vi "PreprocessMotorStages.vi"(3 "Speed Regulation":bool, 5 "Wait":bool=TRUE, 6 "Direction (T: Fwd)":bool=TRUE, 7 "Stop After":bool=TRUE, 8 "Power":i32=75, 9 "Ramp Mode":T5 items=["Constant", "Ramp Up", "Ramp Down"], 10 "Goal":i32=360, 11 "Goal Type":T4=1 items=["Unlimited", "Distance", "Time", "Stop"]) -> (1 "stages":i32=2, 2 "stage definitions":T1[](array[typedef])=[{"Power"=75, "Mode"=3, "RegMode"=0, "RunState"=32, "Goal Type"=1, "Goal"=360, "Update Flags"=39}, {"Power"=0, "Mode"=7, "RegMode"=1, "RunState"=32, "Goal Type"=3, "Goal"=500, "Update Flags"=7}] {"Update Flags" format="%.0x"; "Goal Type" items=["Unlimited", "Distance", "Time", "Stop"]; "RunState" format="%02.0f" items=["IDLE"=0, "RAMPUP"=16, "RUNNING"=32, "RAMPDOWN"=64]; "RegMode" format="%02.0f" items=["IDLE", "SPEED", "SYNC"]; "Mode" format="%.0x"})   [LabVIEW 2009]
uses:
  <vilib>/NXT/Block Support/NXT_Motor.Action.ctl
  <vilib>/NXT/Block Support/NXT_OutputGoalType.ctl
  MotorStageDefinition.ctl
  Move/RegMode.ctl
  Move/RunState.ctl
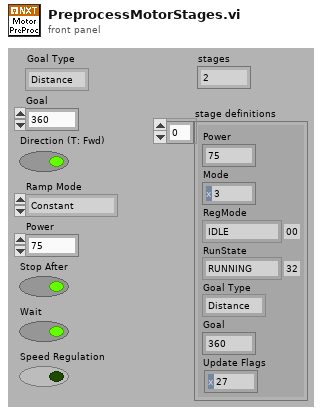
[diagram p1: front panel]
types:
  T1 = typedef "MotorStageDefinition.ctl" = cluster{"Power":i8, "Mode":u8, "RegMode":T2, "RunState":T3, "Goal Type":T4, "Goal":u32, "Update Flags":u8}
  T2 = typedef "RegMode.ctl" = u8
  T3 = typedef "RunState.ctl" = u8
  T4 = typedef "NXT_OutputGoalType.ctl" = u16
  T5 = typedef "NXT_Motor.Action.ctl" = u16
  T6 = cluster{i8, u8, "RegMode":T2, "RunState":T3, "Goal Type":T4, "Goal":u32, u8}
  T7 = cluster{i8, u8, "RegMode":T2, "RunState":T3, u8, "Absolute Value":i32, u8}
  T8 = cluster{i8, u8, "RegMode":T2, "RunState":T3, u8, "Absolute Value":i32, u8}[]
  T9 = cluster{i8, u8, "RegMode":T2, "RunState":T3, "Goal Type":T4, "Goal":u32, u8}[]
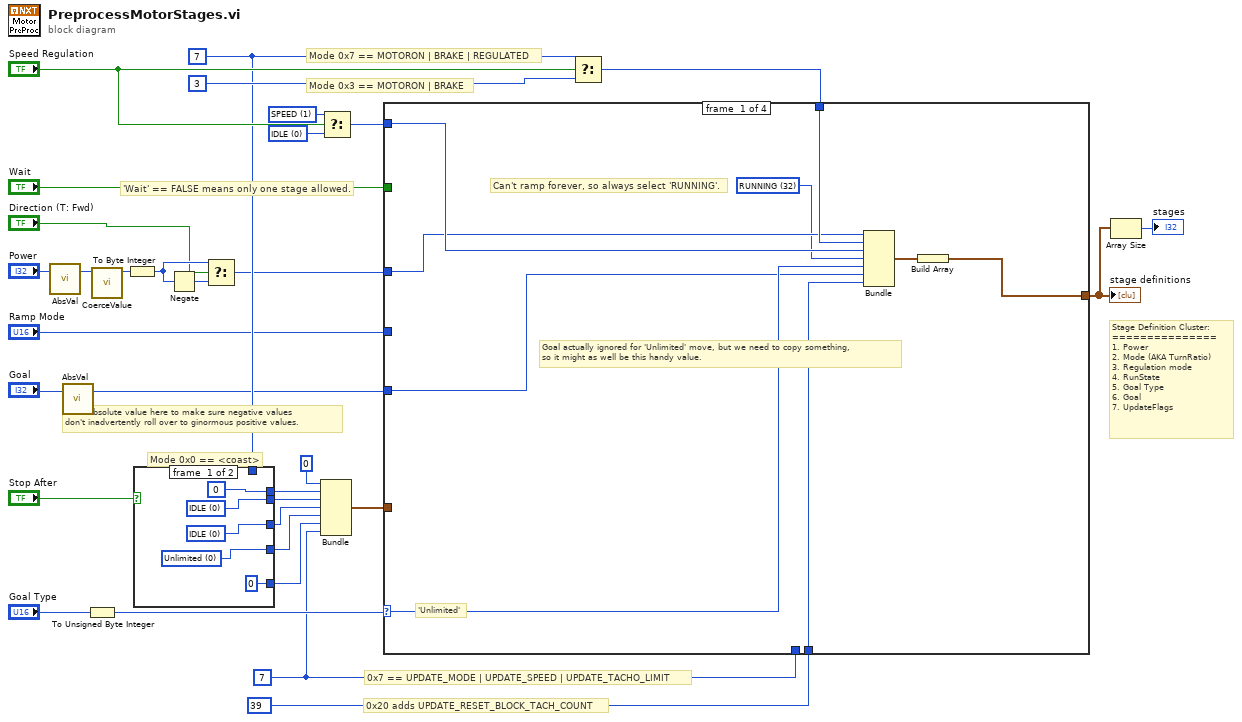
[diagram p0: block diagram]
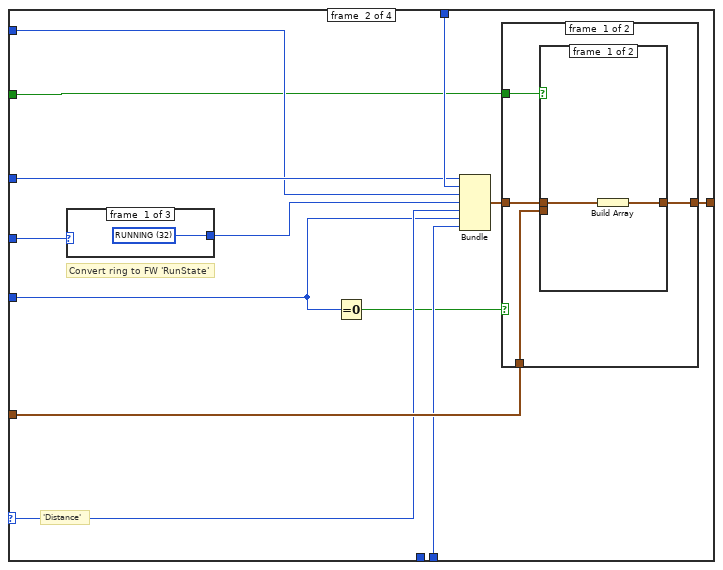
[diagram p2: hidden frame]
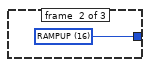
[diagram p3: hidden frame]
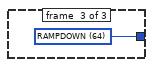
[diagram p4: hidden frame]
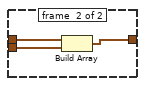
[diagram p5: hidden frame]
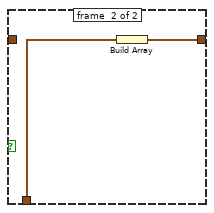
[diagram p6: hidden frame]
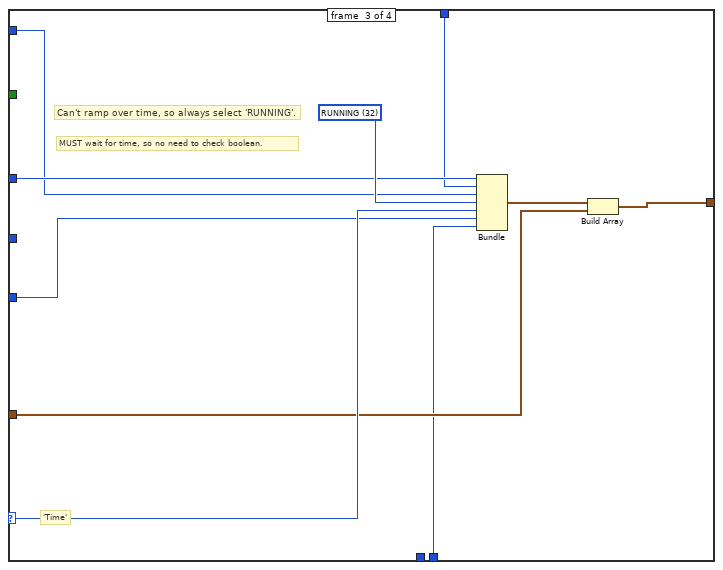
[diagram p7: hidden frame]
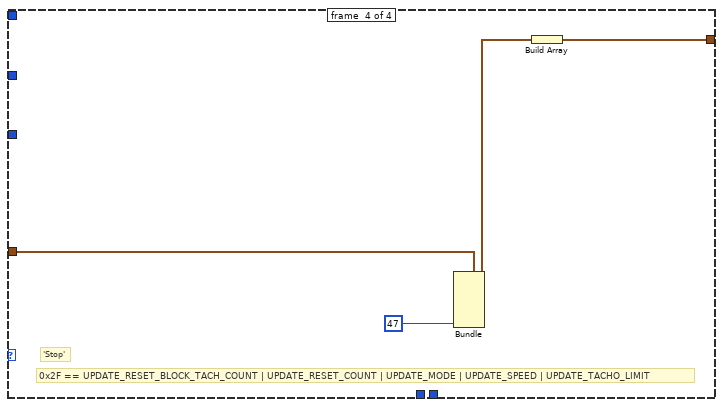
[diagram p8: hidden frame]
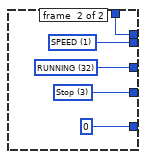
[diagram p9: hidden frame]
diagram:
  w18 = u8 7
  w14 = u8 7
  w25 = T2 1 items=["IDLE", "SPEED", "SYNC"] ("RegMode")
  w26 = T2 0 items=["IDLE", "SPEED", "SYNC"] ("RegMode")
  # "Take absolute value here to make sure negative values\ndon't inadvertently roll over to ginormous positive values."
  # "Mode 0x3 == MOTORON | BRAKE"
  # "Mode 0x7 == MOTORON | BRAKE | REGULATED"
  # "0x20 adds UPDATE_RESET_BLOCK_TACH_COUNT"
  # "0x7 == UPDATE_MODE | UPDATE_SPEED | UPDATE_TACHO_LIMIT"
  # "'Wait' == FALSE means only one stage allowed."
  # "Stage Definition Cluster:\n===============\n1. Power\n2. Mode (AKA TurnRatio)\n3. Regulation mode\n4. RunState\n5. Goal Type\n6. Goal\n7. UpdateFlags"
  n1 = call <vilib>:"AbsVal.vi"("Integer"="Power") -> ("Absolute Value"=w9:i32)  [unwired: 2 in]
  n2 = call <vilib>:"AbsVal.vi"("Integer"="Goal") -> ("Absolute Value"=w6:i32)  [unwired: 2 in]
  n3 = To Unsigned Byte Integer(number="Goal Type") -> (unsigned 8bit integer=w23:u8)
  n4 = call <vilib>:"CoerceValue.vi"("Numeric"=w9) -> ("Numeric Out"=w4:i32)  [unwired: 10 in]
  n5 = To Byte Integer(number=w4) -> (8bit integer=w3:i8)
  n6 = case shown="True" "Stop After" {
    tunnel: [w37 w42] -> w30
    tunnel: [w34 w39] -> w32
    tunnel: [u32 0 ("Goal") u32 0 ("Goal")] -> w29
    tunnel: [w36 w40] -> w28
    tunnel: w14 -> [_ w38]
    tunnel: [u8 0 w38] -> w13
    frame #0 {
      w34 = T2 0 items=["IDLE", "SPEED", "SYNC"] ("RegMode")
      w36 = T4 0 items=["Unlimited", "Distance", "Time", "Stop"] ("Goal Type")
      w37 = T3 0 items=["IDLE"=0, "RAMPUP"=16, "RUNNING"=32, "RAMPDOWN"=64] ("RunState")
      # "Mode 0x0 == <coast>"
    }
    frame #1 {
      w39 = T2 1 items=["IDLE", "SPEED", "SYNC"] ("RegMode")
      w40 = T4 3 items=["Unlimited", "Distance", "Time", "Stop"] ("Goal Type")
      w42 = T3 32 items=["IDLE"=0, "RAMPUP"=16, "RUNNING"=32, "RAMPDOWN"=64] ("RunState")
    }
  }
  n7 = Negate(x=w3) -> (-x=w10:i8)
  n8 = Select(t=w3, s="Direction (T: Fwd)", f=w10) -> (s? t:f=w2:i8)
  n9 = Bundle(i8 0, w13, "RegMode"=w32, "RunState"=w30, "Goal Type"=w28, "Goal"=w29, w18) -> (w21:T6)  [unwired: 1 in]
  n10 = Select(t=w25, s="Speed Regulation", f=w26) -> (s? t:f=w22:T2)
  n11 = Select(t=w14, s="Speed Regulation", f=u8 3) -> (s? t:f=w16:u8)
  n12 = case shown="1" w23 {
    selector: w23 -> [w46 w60 w87 _]
    tunnel: [w51 w59 w80 w92] -> w12
    tunnel: w2 -> [w47 w62 w86 _]
    tunnel: w16 -> [w49 w63 w85 _]
    tunnel: w22 -> [w48 w61 w84 _]
    tunnel: w21 -> [_ w64 w81 w91]
    tunnel: w6 -> [w45 w56 w83 _]
    tunnel: "Wait" -> [_ w57 _ _]
    tunnel: u8 39 -> [w43 w55 w79 _]
    tunnel: w18 -> [_ _ _ _]
    tunnel: "Ramp Mode" -> [_ w53 _ _]
    frame #0 {
      w44 = T3 32 items=["IDLE"=0, "RAMPUP"=16, "RUNNING"=32, "RAMPDOWN"=64] ("RunState")
      # "Can't ramp forever, so always select 'RUNNING'."
      # "'Unlimited'"
      # "Goal actually ignored for 'Unlimited' move, but we need to copy something,\nso it might as well be this handy value."
      n13 = Bundle(w47, w49, "RegMode"=w48, "RunState"=w44, w46, "Absolute Value"=w45, w43) -> (w50:T7)  [unwired: 1 in]
      n14 = Build Array(w50) -> (w51:T8)
    }
    frame #1 {
      # "Convert ring to FW 'RunState'"
      # "'Distance'"
      n15 = case shown="0, Default" w53 {
        tunnel: [w65 w66 w67] -> w52
        frame #0 {
          w65 = T3 32 items=["IDLE"=0, "RAMPUP"=16, "RUNNING"=32, "RAMPDOWN"=64] ("RunState")
        }
        frame #1 {
          w66 = T3 16 items=["IDLE"=0, "RAMPUP"=16, "RUNNING"=32, "RAMPDOWN"=64] ("RunState")
        }
        frame #2 {
          w67 = T3 64 items=["IDLE"=0, "RAMPUP"=16, "RUNNING"=32, "RAMPDOWN"=64] ("RunState")
        }
      }
      n16 = Equal To 0?(x=w56) -> (x = 0?=w54:bool)
      n17 = Bundle(w62, w63, "RegMode"=w61, "RunState"=w52, w60, "Absolute Value"=w56, w55) -> (w58:T7)  [unwired: 1 in]
      n18 = case shown="False" w54 {
        tunnel: w64 -> [w71 w78]
        tunnel: [w70 w77] -> w59
        tunnel: w58 -> [w69 _]
        tunnel: w57 -> [w68 _]
        frame #0 {
          n19 = case shown="False" w68 {
            tunnel: [w72 w76] -> w70
            tunnel: w69 -> [w73 w74]
            tunnel: w71 -> [_ w75]
            frame #0 {
              n20 = Build Array(w73) -> (w72:T8)
            }
            frame #1 {
              n21 = Build Array(w74, w75) -> (w76:T9)
            }
          }
        }
        frame #1 {
          n22 = Build Array(w78) -> (w77:T9)
        }
      }
    }
    frame #2 {
      w88 = T3 32 items=["IDLE"=0, "RAMPUP"=16, "RUNNING"=32, "RAMPDOWN"=64] ("RunState")
      # "MUST wait for time, so no need to check boolean."
      # "Can't ramp over time, so always select 'RUNNING'."
      # "'Time'"
      n23 = Bundle(w86, w85, "RegMode"=w84, "RunState"=w88, w87, "Absolute Value"=w83, w79) -> (w82:T7)  [unwired: 1 in]
      n24 = Build Array(w82, w81) -> (w80:T9)
    }
    frame #3 {
      # "0x2F == UPDATE_RESET_BLOCK_TACH_COUNT | UPDATE_RESET_COUNT | UPDATE_MODE | UPDATE_SPEED | UPDATE_TACHO_LIMIT"
      # "'Stop'"
      n25 = Bundle(cluster=w91, u8 47 ("element")) -> (w90:T6)  [unwired: 6 in]
      n26 = Build Array(w90) -> (w92:T9)
    }
  }
  "stage definitions" <- w12
  n27 = Array Size(array=w12) -> (size(s)=→"stages":i32)
